vi "robotAlignedToLineBallTarget.vi"(4 "DistanceToGoAroundBall":dbl=200.0, 6 "Target":dbl[](array[numeric]), 8 "error in (no error)":errorcluster, 9 "Ball":refnum<class "Ball.lvclass">, 10 "Robot in":refnum<class "Robot.lvclass">, 11 "Utilities in":refnum<class "Utilities.lvclass">) -> (0 "error out":errorcluster, 2 "dest(x, y, orientaion)":dbl[](array[numeric]), 3 "Utilities out":refnum<class "Utilities.lvclass">)   [LabVIEW 2023, in "Utilities.lvclass"]
uses:
  Utilities.lvclass
  Ball_class/Ball.lvclass
  C:/Users/lucio/Desktop/roboime/SSL_AI/Object_class/Object.lvclass
  Robot_class/Robot.lvclass
  Object_class/Object.lvclass/Object.ctl
  <vilib>/Analysis/baseanly.llb/Unit Vector (DBL).vi
  Object_class/Read position(x,y).vi
  <vilib>/Analysis/NI_AALBase.lvlib
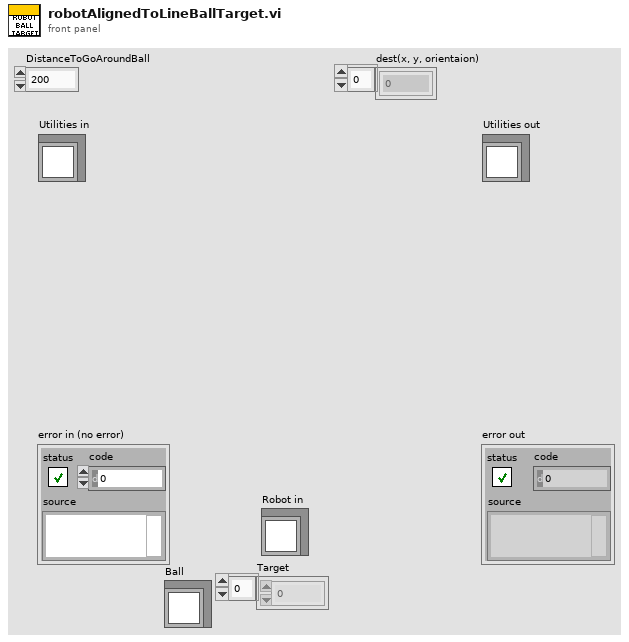
[diagram p1: front panel]
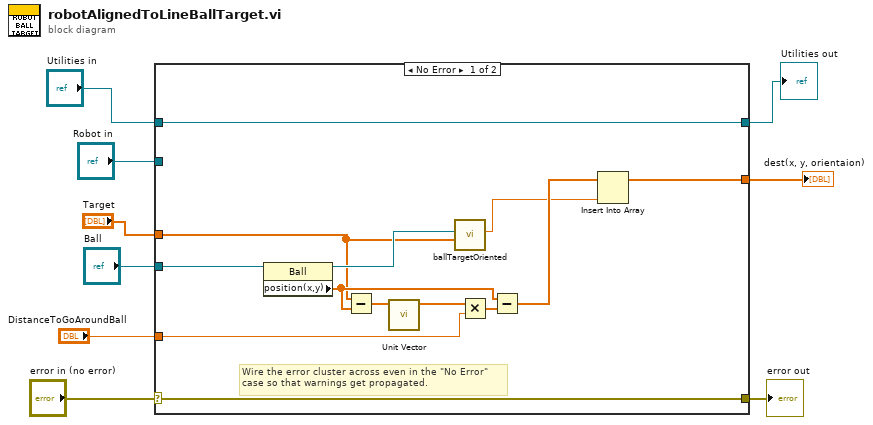
[diagram p0: block diagram]
diagram:
  n1 = case shown="No Error" "error in (no error)" {
    selector: "error in (no error)" -> [w21 w24]
    tunnel: [w21 w24] -> w8
    tunnel: [w22 w23] -> w6
    tunnel: "Utilities in" -> [w22 w23]
    tunnel: "Target" -> [w15 _]
    tunnel: "Ball" -> [w14 _]
    tunnel: "Robot in" -> [_ _]
    tunnel: [w11 _] -> w2
    tunnel: "DistanceToGoAroundBall" -> [w10 _]
    frame No Error {
      # "Wire the error cluster across even in the \"No Error\"\ncase so that warnings get propagated."
      n2 = property class="Ball"(reference=w14) -> (reference out=w17:refnum<class "Ball.lvclass">, "position(x,y)"=w16:dbl[])  [unwired: 1 in, 1 out]
      n3 = Subtract(x=w15, y=w16) -> (x-y=w20:dbl[])
      n4 = call-poly <vilib>:"Unit Vector.vi"("Input Vector"=w20) -> ("Unit Vector"=w19:dbl[])  [unwired: 8 in, 2 out]
      n5 = call "ballTargetOriented.vi"("Target"=w15, "Ball"=w17) -> ("Orientation"=w12:dbl)  [unwired: 7 in, 2 out]
      n6 = Multiply(x=w19, y=w10) -> (x*y=w18:dbl[])
      n7 = Subtract(x=w16, y=w18) -> (x-y=w13:dbl[])
      n8 = Insert Into Array(array=w13, new element=w12) -> (w11:dbl[])  [unwired: 1 in]
    }
    frame Error {
    }
  }
  "error out" <- w8
  "Utilities out" <- w6
  "dest(x, y, orientaion)" <- w2
